vi "Configure Master Wrapper.vi"(8 "error in":errorcluster, 10 "Cyclic Data Bandwidth":u32, 11 "IOV ref in":refnum<k21>) -> (0 "error out":errorcluster, 2 "Cyclic Data Bandwidth out":u32, 3 "IOV ref out":refnum<k21>)   [LabVIEW 2020, in "SEECD Engine.lvlib"]
uses:
  SEECD Engine.lvlib
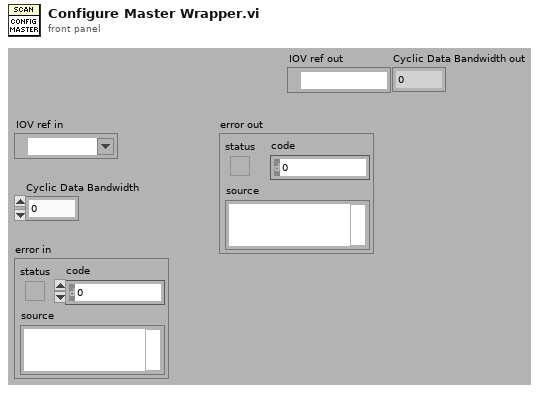
[diagram p1: front panel]
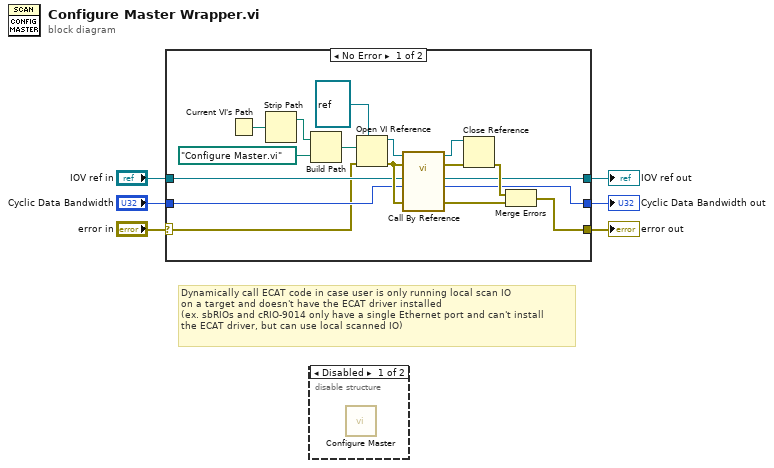
[diagram p0: block diagram]
diagram:
  # "Dynamically call ECAT code in case user is only running local scan IO\non a target and doesn't have the ECAT driver installed\n(ex. sbRIOs and cRIO-9014 only have a single Ethernet port and can't install\nthe ECAT driver, but can use local scanned IO)"
  n1 = case shown="No Error" "error in" {
    selector: "error in" -> [w7 w26]
    tunnel: [w12 w26] -> w6
    tunnel: [w11 w25] -> w5
    tunnel: "Cyclic Data Bandwidth" -> [w10 w25]
    tunnel: "IOV ref in" -> [w9 w24]
    tunnel: [w8 w24] -> w2
    frame No Error {
      n2 = Current VI's Path() -> (path=w14:path)
      n3 = Strip Path(path=w14) -> (stripped path=w16:path)  [unwired: 1 out]
      n4 = Build Path(base path=w16, name or relative path=path "Configure Master.vi" ("vi path")) -> (appended path=w17:path)
      n5 = Open VI Reference(type specifier VI Refnum (for type only)=refnum<vi> refnum, vi path=w17, error in (no error)=w7) -> (vi reference=w19:refnum<vi>, error out=w18:errorcluster)  [unwired: 3 in]
      n6 = call-by-ref "?"(reference=w19, error in=w18, "error in"=w18, "Cyclic Data Bandwidth"=w10, "IOV ref in"=w9) -> (reference out=w21:refnum<vi>, error out=w20:errorcluster, 0:"error out"=w22:errorcluster, "Cyclic Data Bandwidth out"=w11:u32, "IOV ref out"=w8:refnum<k21>)  [unwired: 6 in]
      n7 = Close Reference(reference=w21, error in (no error)=w20) -> (error out=w23:errorcluster)
      n8 = Merge Errors(w23, w22) -> (w12:errorcluster)
    }
    frame Error {
    }
  }
  "error out" <- w6
  "IOV ref out" <- w2
  "Cyclic Data Bandwidth out" <- w5
  n9 = disable-structure shown="Disabled" {
    frame Disabled {
      n10 = call "Configure Master.vi"() -> ()  [unwired: 9 in, 3 out]
    }
    frame Enabled {
    }
  }
